vi "B Sweep T1&Rabi measurements.vi"() -> ()   [LabVIEW 2012]
uses:
  <vilib>/Utility/file.llb/Read From Spreadsheet File (DBL).vi
  <vilib>/Analysis/1siggen.llb/Ramp Pattern by Samples.vi
  <vilib>/Utility/file.llb/Write To Spreadsheet File (DBL).vi
  <vilib>/Analysis/NI_AALBase.lvlib
panel:
  in  "Tab Control":enum32{"T1 ", "T1 2", "Rabi", "T2"}(tab)=enum."Rabi"
  in  "Rest time Min":dbl=5e-08
  in  "Rest time Max":dbl=5e-07
  in  "type":u16(ring) items=["Linear", "Logarithmic"]
  in  "Rest time No. Steps":i32
  in  "samples":i32=128
  in  "end":dbl=1.0 format="%0.2f"
  in  "start":dbl format="%0.2f"
  in  "Tau Max":dbl=0.001
  in  "Tau Min":dbl=2e-08
  in  "Tau No. Steps":i32=20
  in  "type 2":u16(ring)=1 items=["Linear", "Logarithmic"]
  in  "T1 Signal Delay":dbl=6e-07
  in  "T1 APD width":dbl=5e-07
  in  "T1 AOM length":dbl=2.5e-06
  in  "T1 AOM Rest":dbl=1e-06
  in  "ODMR Res/Rabi File":path=path "C:/Users/Ouyang Group/Documents/Data/6-1-16/Dot 1 5mW local ODMR B freq min"
  in  "Pi Pulse?":bool
  in  "MW width Min":dbl=2e-08
  in  "MW width Max":dbl=5e-07
  in  "MW width step size":dbl=5e-09
  in  "MW Delay":dbl=5e-08
  in  "ODMR res file":path
  in  "p (dbm)":dbl
  in  "ODMR Res/Rabi File 2":path=path "C:/Users/Ouyang Group/Documents/Data/6-1-16/Dot 1 5mW local ODMR B freq min"
  in  "p (dbm) 2":dbl
  in  "Tau min":dbl
  in  "Tau max":dbl
  in  "Tau step size":dbl
  in  "Pulse offset":dbl
  in  "MW Delay 2":dbl
  in  "RS232 settings":cluster{"Portnumber":i32, "Baudrate":u16}={"Portnumber"=12, "Baudrate"=5} {"Portnumber" items=["COM1", "COM2", "COM3", "COM4", "COM5", "COM6", "COM7", "COM8", "COM9", "COM10", "COM11", "COM12", "COM13", "COM14", "COM15", "COM16", "COM17", "COM18", "COM19", "COM20", "COM21", "COM22", "COM23", "COM24", "COM25", "COM26", "COM27", "COM28", "COM29", "COM30"]; "Baudrate" items=["9600", "14400", "19200", "38400", "57600", "115200"]}
  in  "Z Pos":dbl
  in  "Y pos":dbl
  in  "X Pos":dbl
  in  "Y Parameters":T1={"Number of Y Steps"=200, "Max Y (V)"=2.0, "Min Y (V)"=-2.0}
  in  "X":T2={"Number of X Steps"=200, "Max X (V)"=2.0, "Min X (V)"=-2.0}
  out "Tracking Loop":dbl=6.0
  in  "N Loop":i32=100000
  in  "ref?":bool=TRUE
  in  "Sig/Ref pause":dbl=5e-07
  in  "APD signal width":dbl=3e-07
  in  "AOM Pulse length":dbl=2.5e-06
  in  "Signal delay":dbl=7.6e-07
  in  "AOM Rest time":dbl=1e-06
  in  "Path to spinapi.dll":path=path "C:/SpinCore/SpinAPI/dll/spinapi64.dll"
  in  "Scan Interval (sec)":dbl=150.0
  in  "Collection Time (sec)":dbl=600.0
  in  "File Path Control":path
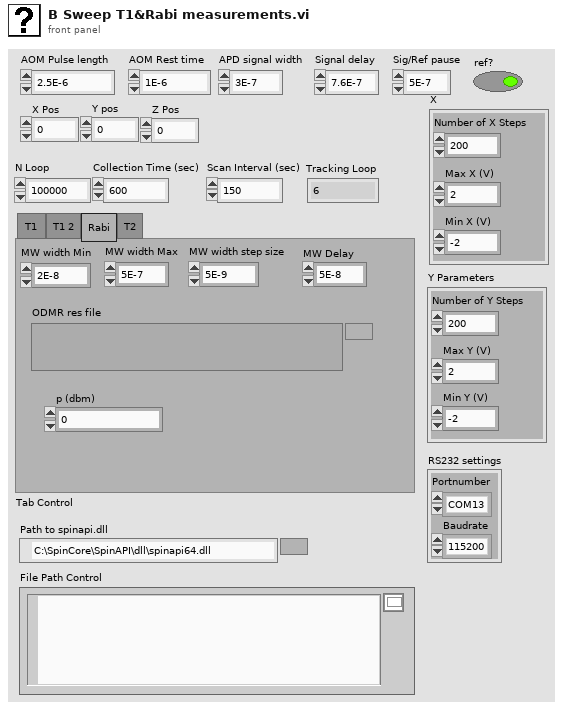
[diagram p1: front panel]
types:
  T1 = cluster{"Number of Y Steps":i32, "Max Y (V)":dbl, "Min Y (V)":dbl}
  T2 = cluster{"Number of X Steps":i32, "Max X (V)":dbl, "Min X (V)":dbl}
  T3 = enum16{"Stop", "Track", "EPR", "Load Pulse Sequence"}
  T4 = cluster{"Instruct Data":i32, "Op Code":i32, "Flags":bool[], "Comments":string, "Time (s)":dbl}
  T5 = enum16{"Pulse Program", "Frequency Registers", "TX Phase Registers", "RX Phase Registers"}
  T6 = cluster{"Instruct Data":i32, "Op Code":i32, "Flags":bool[], "Comments":string, "Time (s)":dbl}[]
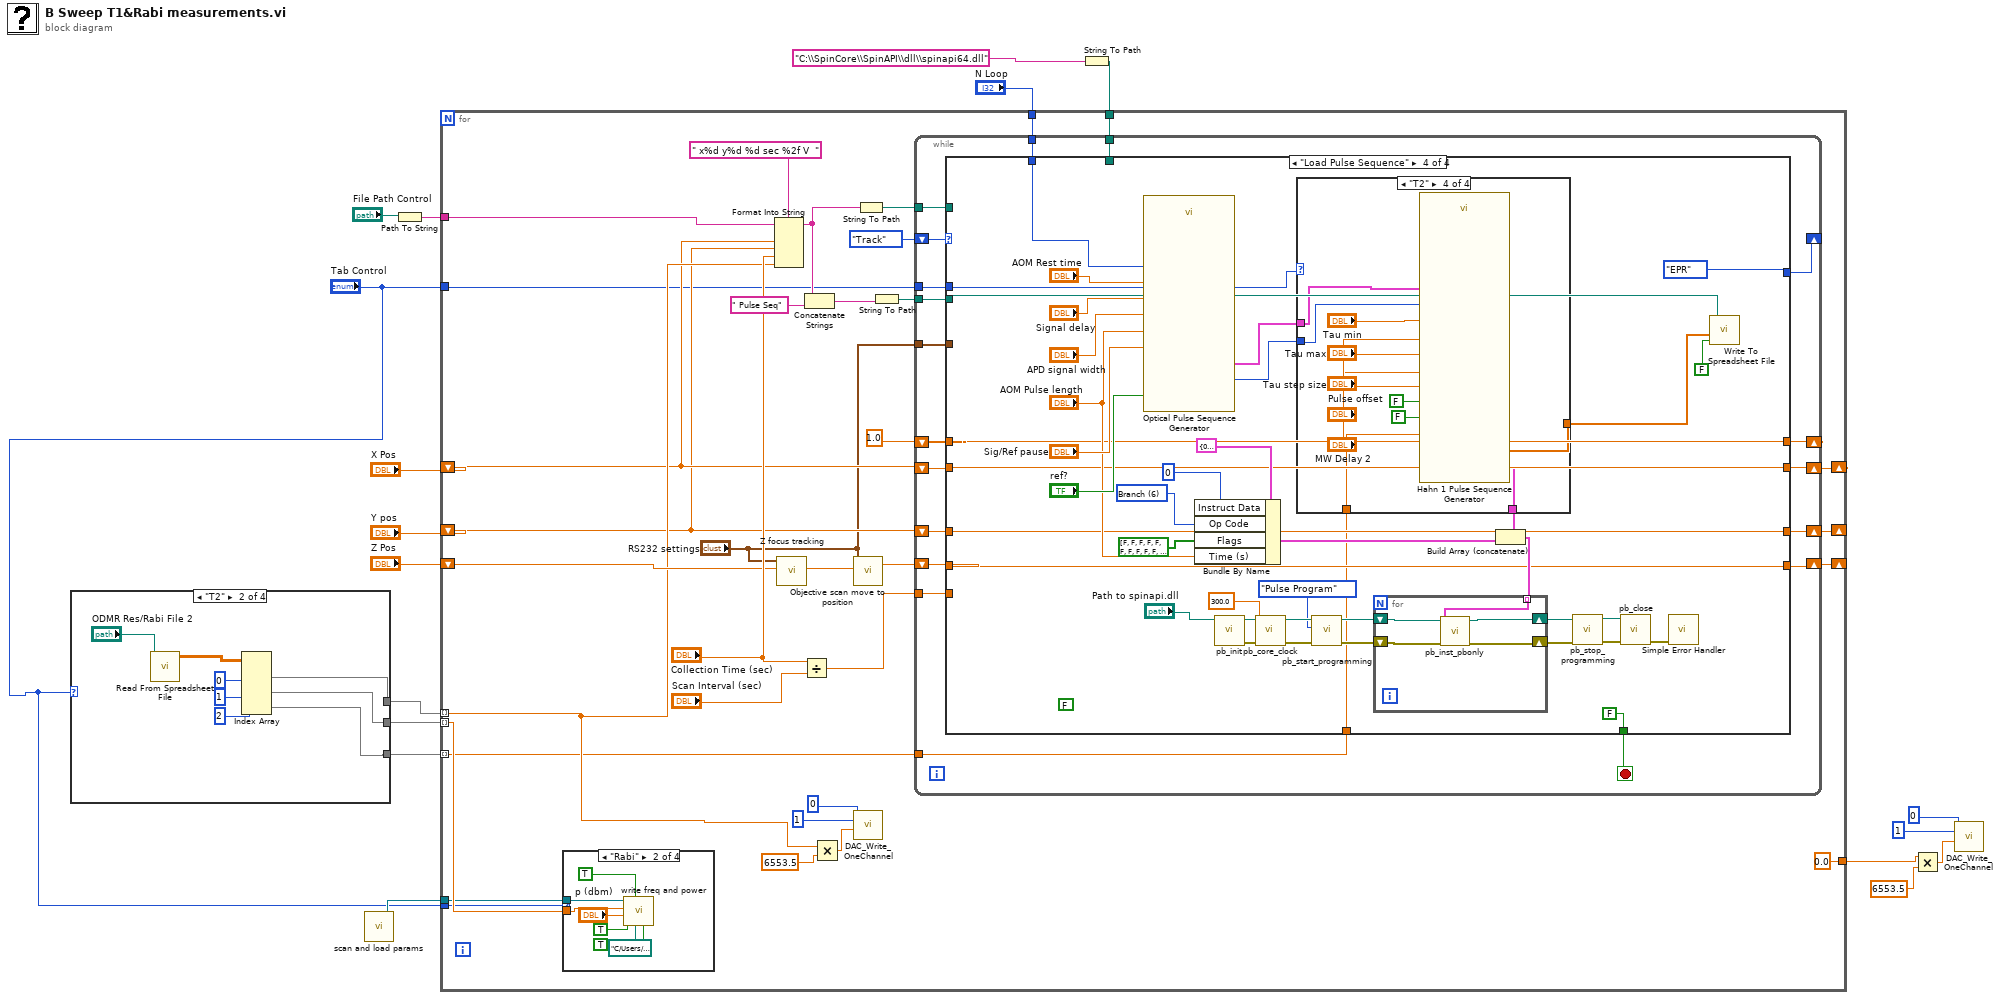
[diagram p0: block diagram]
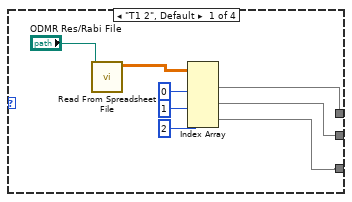
[diagram p2: hidden frame]
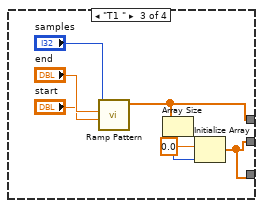
[diagram p3: hidden frame]
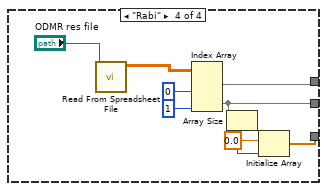
[diagram p4: hidden frame]
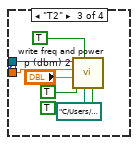
[diagram p6: hidden frame]
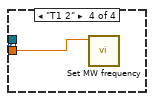
[diagram p7: hidden frame]
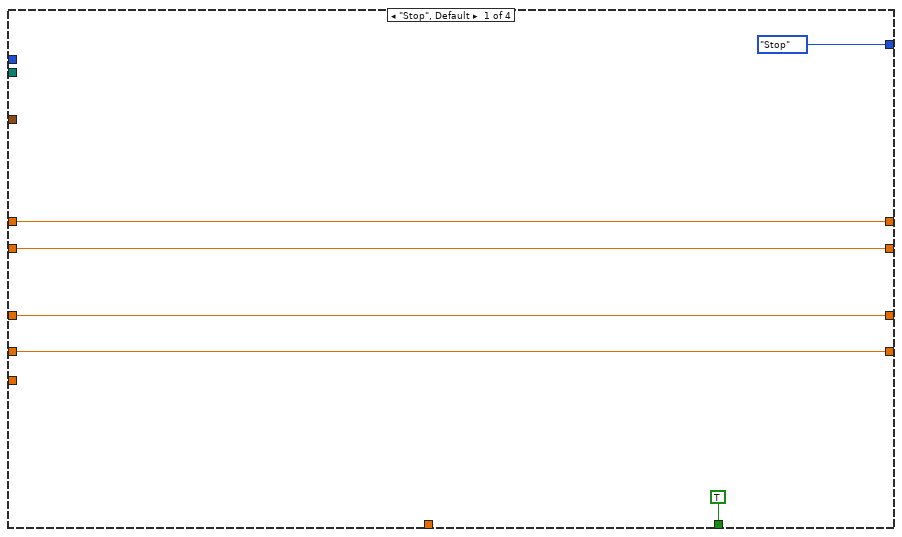
[diagram p8: hidden frame]
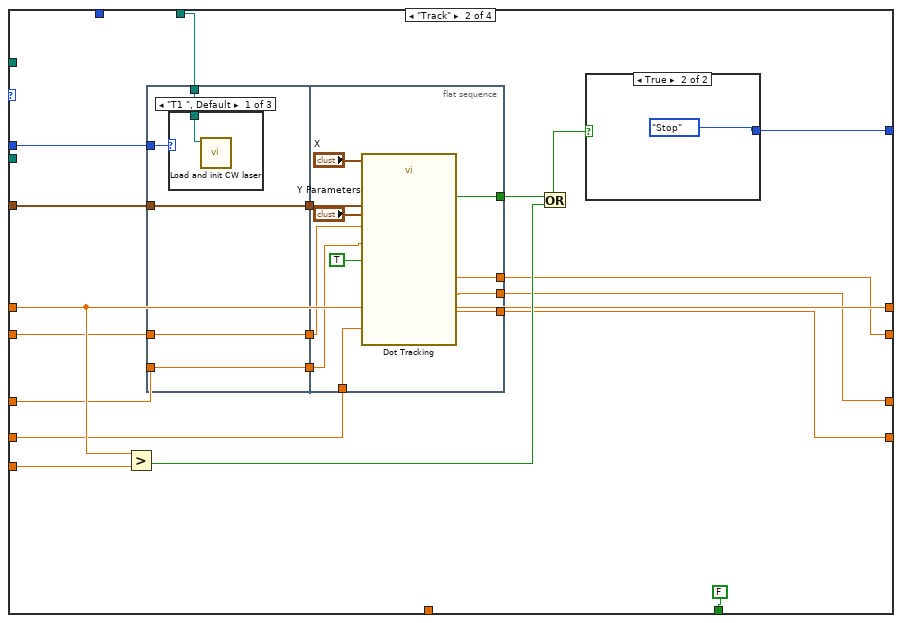
[diagram p9: hidden frame]
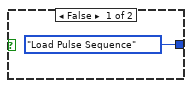
[diagram p10: hidden frame]
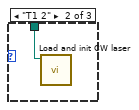
[diagram p11: hidden frame]
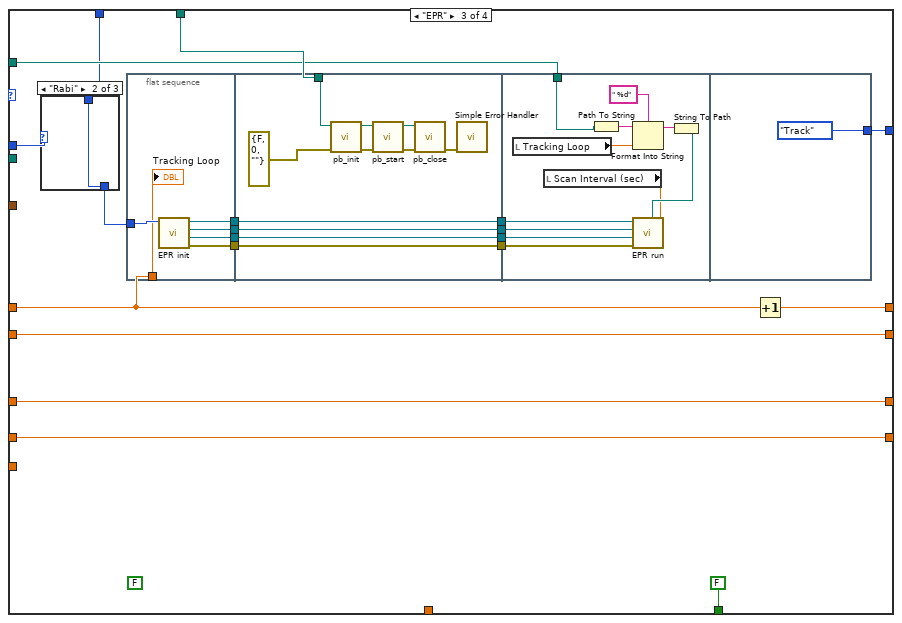
[diagram p13: hidden frame]
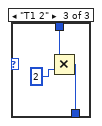
[diagram p15: hidden frame]
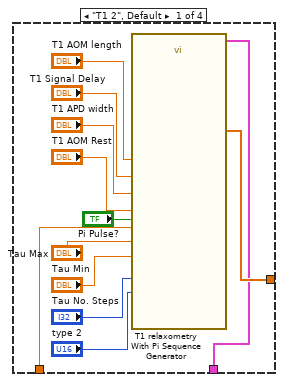
[diagram p16: hidden frame]
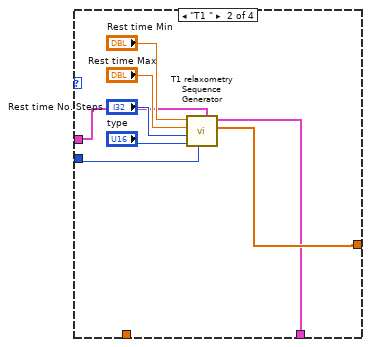
[diagram p17: hidden frame]
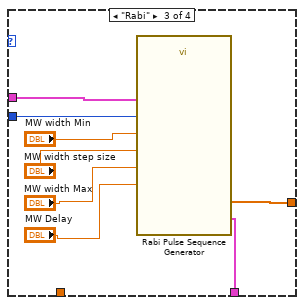
[diagram p18: hidden frame]
diagram:
  n1 = case shown="\"T2\"" "Tab Control" {
    tunnel: [w22 w30 w36 w46] -> w4
    tunnel: [w21 w29 w35 w45] -> w5
    tunnel: [w20 w28 w35 w43] -> w3
    frame "T1 2", Default {
      n2 = call-poly <vilib>:"Read From Spreadsheet File.vi"("file path (dialog if empty)"="ODMR Res/Rabi File") -> ("all rows"=w25:dbl[][])  [unwired: 6 in, 4 out]
      n3 = Index Array(array=w25, index (col) #1=0 ("disabled index (col)"), index (col) #2=1 ("index (col)"), index (col) #3=2 ("index (col)")) -> (element #1=w22:dbl[], element #2=w21:dbl[], element #3=w20:dbl[])  [unwired: 3 in]
    }
    frame "T2" {
      n4 = call-poly <vilib>:"Read From Spreadsheet File.vi"("file path (dialog if empty)"="ODMR Res/Rabi File 2") -> ("all rows"=w33:dbl[][])  [unwired: 6 in, 4 out]
      n5 = Index Array(array=w33, index (col) #1=0 ("disabled index (col)"), index (col) #2=1 ("index (col)"), index (col) #3=2 ("index (col)")) -> (element #1=w30:dbl[], element #2=w29:dbl[], element #3=w28:dbl[])  [unwired: 3 in]
    }
    frame "T1 " {
      n6 = call-poly <vilib>:"Ramp Pattern.vi"("start"="start", "end"="end", "samples"="samples") -> ("Ramp Pattern"=w36:dbl[])  [unwired: 7 in, 1 out]
      n7 = Array Size(array=w36) -> (size(s)=w38:i32)
      n8 = Initialize Array(0.0 ("element"), w38) -> (w35:dbl[])
    }
    frame "Rabi" {
      n9 = call-poly <vilib>:"Read From Spreadsheet File.vi"("file path (dialog if empty)"="ODMR res file") -> ("all rows"=w49:dbl[][])  [unwired: 6 in, 4 out]
      n10 = Index Array(array=w49, index (col) #1=0 ("disabled index (col)"), index (col) #2=1 ("index (col)")) -> (element #1=w46:dbl[], element #2=w45:dbl[])  [unwired: 2 in]
      n11 = Array Size(array=w45) -> (size(s)=w44:i32)
      n12 = Initialize Array(0.0 ("element"), w44) -> (w43:dbl[])
    }
  }
  n13 = call "scan and load params.vi"() -> ("Serial Port Select"=w2:refnum<visa-resource-name>)  [unwired: 9 out]
  n14 = Path To String(path="File Path Control") -> (string=w17:string)
  n15 = String To Path(string="C:\\SpinCore\\SpinAPI\\dll\\spinapi64.dll") -> (path=w15:path)
  n16 = for {
    shift-right: [w79] -> _
    shift-left: "X Pos" -> [w63]
    shift-right: [w78] -> _
    shift-left: "Y pos" -> [w62]
    tunnel: w17 -> [w84]
    tunnel: w15 -> [w81]
    tunnel: "N Loop" -> [w77]
    tunnel: w4 -> [w64] mode=indexing
    shift-right: [w68] -> _
    shift-left: "Z Pos" -> [w66]
    tunnel: [0.0 ("x")] -> w6
    tunnel: "Tab Control" -> [w59]
    tunnel: w5 -> [w58] mode=indexing
    tunnel: w3 -> [w57] mode=indexing
    tunnel: "Tab Control" -> [w52]
    tunnel: w2 -> [w51]
    n17 = case shown="\"Rabi\"" w52 {
      tunnel: w58 -> [_ w91 w98 w99]
      tunnel: w51 -> [_ w90 w97 _]
      frame "T1 ", Default {
      }
      frame "Rabi" {
        n18 = call "write freq and power.vi"("leveling"=TRUE, "leviling file"=path "C:/Users/Ouyang Group/Documents/Data/8-26-16/Windfreak plus switches and amp power calibration high res", "Channel"=TRUE, "RF On"=TRUE, "p (dbm)"="p (dbm)", "f (Hz)"=w91, "Serial Port Select"=w90) -> ()  [unwired: 3 in, 2 out]
      }
      frame "T2" {
        n19 = call "write freq and power.vi"("leveling"=TRUE, "leviling file"=path "C:/Users/Ouyang Group/Documents/Data/8-26-16/Windfreak plus switches and amp power calibration high res", "Channel"=TRUE, "RF On"=TRUE, "p (dbm)"="p (dbm) 2", "f (Hz)"=w98, "Serial Port Select"=w97) -> ()  [unwired: 3 in, 2 out]
      }
      frame "T1 2" {
        n20 = call "Set MW frequency.vi"("freq"=w99) -> ()  [unwired: 8 in, 3 out]
      }
    }
    n21 = Format Into String(format string=" x%d y%d %d sec %2f V  ", initial string=w84, w63, w62, "Collection Time (sec)", w64) -> (resulting string=w76:string)  [unwired: 1 in, 1 out]
    n22 = call "Z focus tracking.vi"("Position"=w66, "RS232 settings"="RS232 settings") -> ("center"=w67:dbl)  [unwired: 6 in, 2 out]
    n23 = Divide(x="Collection Time (sec)", y="Scan Interval (sec)") -> (x/y=w70:dbl)
    n24 = Concatenate Strings(w76, " Pulse Seq" ("string")) -> (w74:string)
    n25 = Multiply(x=w64, y=6553.5) -> (x*y=w56:dbl)
    n26 = call "Objective scan move to position.vi"("Z position"=w67, "RS232 settings"="RS232 settings") -> ("Z Position 2"=w65:dbl)  [unwired: 9 in]
    n27 = call "DAC_Write_OneChannel.vi"("Value"=w56, "Channel"=u16 1, "DeviceIndex"=u64 0) -> ()  [unwired: 7 in, 2 out]
    n28 = String To Path(string=w76) -> (path=w75:path)
    n29 = String To Path(string=w74) -> (path=w73:path)
    n30 = while {
      tunnel: w81 -> [w118]
      shift-right: [w116] -> w79
      shift-left: w63 -> [w115]
      shift-right: [w117] -> w78
      shift-left: w62 -> [w114]
      shift-right: [w111] -> _
      shift-left: T3."Track" -> [w113]
      tunnel: w77 -> [w110]
      tunnel: w75 -> [w109]
      tunnel: w73 -> [w108]
      shift-right: [w106] -> _
      shift-left: 1.0 -> [w107]
      tunnel: w70 -> [w105]
      shift-right: [w103] -> w68
      shift-left: w65 -> [w104]
      tunnel: "RS232 settings" -> [w102]
      tunnel: w59 -> [w101]
      tunnel: w57 -> [w100]
      stop <- w112 stop-if-true
      n31 = case shown="\"Load Pulse Sequence\"" w113 {
        tunnel: w118 -> [_ w143 w175 _]
        tunnel: [w121 w134 w173 w222] -> w116
        tunnel: [w120 w133 w169 w221] -> w117
        tunnel: w115 -> [w121 w130 w173 w222]
        tunnel: w114 -> [w120 w128 w169 w221]
        tunnel: [T3."Stop" w141 w170 T3."EPR"] -> w111
        tunnel: [TRUE FALSE FALSE FALSE] -> w112
        tunnel: w110 -> [_ _ w165 w226]
        tunnel: w109 -> [_ _ w174 _]
        tunnel: w108 -> [_ _ _ w225]
        tunnel: w107 -> [w122 w136 w168 w223]
        tunnel: [w122 w136 w171 w223] -> w106
        tunnel: w105 -> [_ w139 _ _]
        tunnel: w104 -> [w119 w135 w167 w220]
        tunnel: [w119 w132 w167 w220] -> w103
        tunnel: w102 -> [_ w127 _ _]
        tunnel: w101 -> [_ w125 w166 w219]
        tunnel: w100 -> [_ _ _ w218]
        frame "Stop", Default {
        }
        frame "Track" {
          n32 = Greater?(x=w136, y=w139) -> (0:w137:bool)
          n33 = flat-sequence {
            tunnel: w143 -> [w150]
            tunnel: [w149] -> w131
            tunnel: w130 -> [w149]
            tunnel: [w148] -> w129
            tunnel: w128 -> [w148]
            tunnel: w127 -> [w147]
            tunnel: [w147] -> w126
            tunnel: w125 -> [w146]
            tunnel: [w163] -> w134
            tunnel: [w162] -> w133
            tunnel: [w160] -> w142
            tunnel: w135 -> [w157]
            tunnel: [w156] -> w132
            tunnel: w131 -> [w155]
            tunnel: w129 -> [w154]
            tunnel: w126 -> [w153]
            frame #0 {
              n34 = case shown="\"T1 \", Default" w146 {
                tunnel: w150 -> [w151 w152 _]
                frame "T1 ", Default {
                  n35 = call "Load and init CW laser.vi"("path in"=w151) -> ()  [unwired: 11 in]
                }
                frame "T1 2" {
                  n36 = call "Load and init CW laser.vi"("path in"=w152) -> ()  [unwired: 11 in]
                }
                frame "Rabi" {
                }
              }
            }
            frame #1 {
              n37 = call "Dot Tracking.vi"("X"="X", "Y Parameters"="Y Parameters", "RS232 settings"=w153, "X Pos"=w155, "Y pos"=w154, "Z Pos"=w157, "Z-track?"=TRUE) -> ("X Position"=w163:dbl, "Y Position"=w162:dbl, "Z Position"=w156:dbl, "Gave up?"=w160:bool)  [unwired: 2 in, 3 out]
            }
          }
          n38 = Or(x=w142, y=w137) -> (x .or. y?=w138:bool)
          n39 = case shown="True" w138 {
            tunnel: [T3."Load Pulse Sequence" T3."Stop"] -> w141
            frame False {
            }
            frame True {
            }
          }
        }
        frame "EPR" {
          (unwired) FALSE
          n40 = case shown="\"Rabi\"" w166 {
            tunnel: w165 -> [w184 w185 w188]
            tunnel: [w184 w185 w186] -> w164
            frame "T1 ", Default {
            }
            frame "Rabi" {
            }
            frame "T1 2" {
              n41 = Multiply(x=w188, y=2) -> (x*y=w186:i32)
            }
          }
          n42 = flat-sequence {
            tunnel: [w194] -> w183
            tunnel: [w193] -> w182
            tunnel: [w192] -> w181
            tunnel: [w191] -> w180
            tunnel: w164 -> [w190]
            tunnel: w168 -> [w189]
            tunnel: [w199] -> w179
            tunnel: w183 -> [w199]
            tunnel: [w198] -> w178
            tunnel: w182 -> [w198]
            tunnel: [w197] -> w177
            tunnel: w181 -> [w197]
            tunnel: [w196] -> w176
            tunnel: w180 -> [w196]
            tunnel: w175 -> [w195]
            tunnel: w179 -> [w210]
            tunnel: w178 -> [w209]
            tunnel: w177 -> [w208]
            tunnel: w176 -> [w207]
            tunnel: w174 -> [w206]
            tunnel: [T3."Track"] -> w170
            frame #0 {
              n43 = call "EPR init.vi"("N loops"=w190) -> ("error out"=w191:errorcluster, "ref task out"=w192:refnum<k21>, "sig task out"=w193:refnum<k21>, "clock task out"=w194:refnum<k21>)  [unwired: 7 in]
              "Tracking Loop" <- w189
            }
            frame #1 {
              n44 = call "pb_init.vi"("error in (no error)"=errorcluster {"status"=FALSE, "code"=0, "source"=""}, "path in"=w195) -> ("error out"=w203:errorcluster, "path out"=w201:path)  [unwired: 1 in, 7 out]
              n45 = call "pb_start.vi"("error in (no error)"=w203, "path in"=w201) -> ("error out"=w204:errorcluster, "path out"=w200:path)  [unwired: 1 in, 7 out]
              n46 = call "pb_close.vi"("error in (no error)"=w204, "path in"=w200) -> ("error out"=w205:errorcluster)  [unwired: 9 out]
              n47 = call <vilib>:"Simple Error Handler.vi"("error in (no error)"=w205) -> ()  [unwired: 1 in, 8 out]
            }
            frame #2 {
              n48 = local read "Tracking Loop"() -> (w213:dbl)
              n49 = local read "Scan Interval (sec)"() -> (w211:dbl)
              n50 = Path To String(path=w206) -> (string=w215:string)
              n51 = Format Into String(format string=" %d", initial string=w215, w213) -> (resulting string=w214:string)  [unwired: 1 in, 1 out]
              n52 = String To Path(string=w214) -> (path=w212:path)
              n53 = call "EPR run.vi"("control task in"=w210, "sig task in"=w209, "ref task in"=w208, "error in"=w207, "file path (dialog if empty)"=w212, "Measurement Interval"=w211) -> ()  [unwired: 4 in]
            }
            frame #3 {
            }
          }
          n54 = Increment(x=w168) -> (x+1=w171:dbl)
        }
        frame "Load Pulse Sequence" {
          (unwired) FALSE
          w252 = 6 items=["Continue", "Stop", "Loop", "End Loop", "JSR", "RTS", "Branch", "Long Delay", "Wait"] ("Op Code")
          n55 = call "Optical Pulse Sequence Generator.vi"("ref?"="ref?", "N Loop"=w226, "Sig/Ref pause"="Sig/Ref pause", "AOM Rest time"="AOM Rest time", "Signal delay"="Signal delay", "APD signal width"="APD signal width", "AOM Pulse length"="AOM Pulse length") -> ("Array"=w233:T6, "No. Instructions"=w232:i32)  [unwired: 3 in]
          n56 = Bundle By Name(cluster=T4 {"Instruct Data"=0, "Op Code"=0, "Flags"=[FALSE, FALSE, FALSE, FALSE, FALSE, FALSE, FALSE, FALSE, FALSE, FALSE, FALSE, FALSE, FALSE, FALSE, FALSE, FALSE, FALSE, FALSE, FALSE, FALSE, FALSE, TRUE, TRUE, TRUE], "Comments"="", "Time (s)"=0.01} ("PB Inst 2"), "Instruct Data"=0, "Op Code"=w252, "Flags"=bool[] [FALSE, FALSE, FALSE, FALSE, FALSE, FALSE, FALSE, FALSE, FALSE, FALSE, FALSE, FALSE, FALSE, FALSE, FALSE, FALSE, FALSE, FALSE, FALSE, FALSE, FALSE, TRUE, TRUE, TRUE], "Time (s)"="AOM Pulse length") -> (w230:T4)
          n57 = call "pb_init.vi"("path in"="Path to spinapi.dll") -> ("error out"=w241:errorcluster, "path out"=w239:path)  [unwired: 3 in, 6 out]
          n58 = call "pb_core_clock.vi"("error in (no error)"=w241, "clock_freq (MHz)"=300.0, "path in"=w239) -> ("error out"=w242:errorcluster, "path out"=w240:path)  [unwired: 7 in]
          n59 = case shown="\"T2\"" w219 {
            tunnel: w233 -> [_ w273 w286 w298]
            tunnel: w232 -> [_ w278 w285 w297]
            tunnel: [w261 w271 w284 w288] -> w231
            tunnel: [w262 w272 w283 w287] -> w228
            tunnel: w218 -> [w260 _ _ w289]
            frame "T1 2", Default {
              n60 = call "T1 relaxometry With Pi Sequence Generator.vi"("AOM Pulse length"="T1 AOM length", "AOM Rest time"="T1 AOM Rest", "Signal Delay"="T1 Signal Delay", "APD signal width"="T1 APD width", "Rabi Freq"=w260, "Pi Pulse?"="Pi Pulse?", "Tau Min"="Tau Min", "Tau Max"="Tau Max", "Tau No. Steps"="Tau No. Steps", "type"="type 2") -> ("Array"=w261:T6, "Tau Pattern"=w262:dbl[])  [unwired: 8 in]
            }
            frame "T1 " {
              n61 = call "T1 relaxometry Sequence Generator.vi"("Optical Pulse"=w273, "No. Instructions"=w278, "type"="type", "Rest time No. Steps"="Rest time No. Steps", "Rest time Max"="Rest time Max", "Rest time Min"="Rest time Min") -> ("Pulse Width"=w272:dbl[], "Pulse Sequence Out"=w271:T6)  [unwired: 4 in]
            }
            frame "Rabi" {
              n62 = call "Rabi Pulse Sequence Generator.vi"("Optical Pulse"=w286, "No. Instructions"=w285, "MW Delay"="MW Delay", "MW width step size"="MW width step size", "MW width Max"="MW width Max", "MW width Min"="MW width Min") -> ("Pulse Width"=w283:dbl[], "Pulse Sequence Out"=w284:T6)  [unwired: 4 in]
            }
            frame "T2" {
              n63 = call "Hahn 1 Pulse Sequence Generator.vi"("Pulse offset"="Pulse offset", "Extra Pi?"=FALSE, "Equal Pulse length"=FALSE, "Array"=w298, "MW Delay"="MW Delay 2", "No. Instructions"=w297, "Tau step size"="Tau step size", "Tau max"="Tau max", "Tau min"="Tau min", "Rabi Frequency"=w289) -> ("Tau"=w287:dbl[], "Pulse Sequence"=w288:T6)
            }
          }
          n64 = call "pb_start_programming.vi"("error in (no error)"=w242, "Device"=T5."Pulse Program", "path in"=w240) -> ("error out"=w245:errorcluster, "path out"=w244:path)  [unwired: 1 in, 6 out]
          n65 = Build Array (concatenate)(w231, w230) -> (w229:T6)
          n66 = for {
            shift-right: [w301] -> w246
            shift-left: w244 -> [w303]
            shift-right: [w300] -> w247
            shift-left: w245 -> [w302]
            tunnel: w229 -> [w299] mode=indexing
            n67 = call "pb_inst_pbonly.vi"("error in (no error)"=w302, "PB Instruction"=w299, "path in"=w303) -> ("error out"=w300:errorcluster, "path out"=w301:path)  [unwired: 2 in, 5 out]
          }
          n68 = call "pb_stop_programming.vi"("error in (no error)"=w247, "path in"=w246) -> ("error out"=w238:errorcluster, "path out"=w237:path)  [unwired: 1 in, 7 out]
          n69 = call "pb_close.vi"("error in (no error)"=w238, "path in"=w237) -> ("error out"=w249:errorcluster)  [unwired: 9 out]
          n70 = call <vilib>:"Simple Error Handler.vi"("error in (no error)"=w249) -> ()  [unwired: 1 in, 8 out]
          n71 = call-poly <vilib>:"Write To Spreadsheet File.vi"("transpose? (no:F)"=FALSE, "1D data"=w228, "file path (dialog if empty)"=w225) -> ()  [unwired: 5 in, 1 out]
        }
      }
    }
  }
  n72 = Multiply(x=w6, y=6553.5) -> (x*y=w9:dbl)
  n73 = call "DAC_Write_OneChannel.vi"("Value"=w9, "Channel"=u16 1, "DeviceIndex"=u64 0) -> ()  [unwired: 7 in, 2 out]
